vi "CreateWaveData.vi"(8 "error in (no error)":errorcluster, 11 "WaveGenerator in":refnum<class "WaveGenerator.lvclass">) -> (0 "error out":errorcluster, 2 "signal out":waveform(dbl), 3 "WaveGenerator out":refnum<class "WaveGenerator.lvclass">)   [LabVIEW 2017, in "WaveGenerator.lvclass"]
uses:
  WaveGenerator.lvclass
  <vilib>/measure/NI_MABase.lvlib
  <vilib>/addons/_Workers/Library/Classes/Worker/Worker.lvclass
  <vilib>/addons/_Workers/Library/Classes/Worker/Read ID.vi
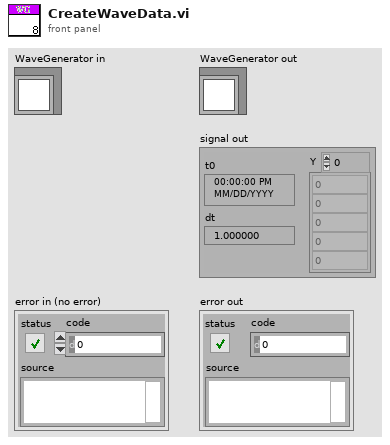
[diagram p1: front panel]
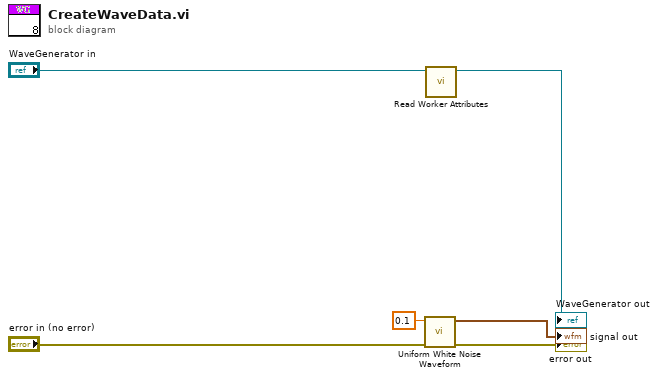
[diagram p0: block diagram]
diagram:
  n1 = call <vilib>:"Uniform White Noise Waveform.vi"("error in (no error)"="error in (no error)", "amplitude"=0.1 ("frequency")) -> ("error out"=→"error out":errorcluster, "signal out"=→"signal out":waveform(dbl))  [unwired: 8 in]
  n2 = call-poly <vilib>:"Read Worker Attributes.vi"("Worker"="WaveGenerator in") -> ("dup Worker out"=→"WaveGenerator out":refnum<class "WaveGenerator.lvclass">)  [unwired: 9 in, 1 out]
